vi "VectorLength.vi"(1 "VectorIn":T1) -> (0 "VectorLength":dbl)   [LabVIEW 2017]
uses:
  PathPlanning/TypeDefs/Point2D.ctl
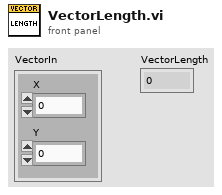
[diagram p1: front panel]
types:
  T1 = typedef "Point2D.ctl" = cluster{"X":dbl, "Y":dbl}
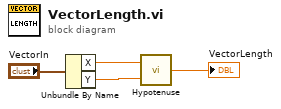
[diagram p0: block diagram]
diagram:
  n1 = Unbundle By Name("VectorIn") -> ("X"=w3:dbl, "Y"=w2:dbl)
  n2 = call "Hypotenuse.vi"("Y"=w2, "X"=w3) -> ("Hypotenuse"=→"VectorLength":dbl)
